vi "FRCts20_Backend_IssueTeamList.vi"(8 "error in (no error)":errorcluster) -> (0 "error out":errorcluster, 2 "IssueTeamList":T1)   [LabVIEW 2013, in "FRCts20_Backend_WebMethods.lvlib"]
doc: "The IssueTeamList function returns all teams with a currently open issue. It is sorted by open time longest to shortest. Caller is provided <b>Open time</b>, <b>Team Number</b>, <b>Loacation</b>, and <b>Description</b>."
uses:
  FRCts20_Backend_WebMethods.lvlib
  FRCts20_Backend_FGVOperation.ctl
  FRCts20_Backend_Engine.lvlib
  FRCts20_Backend_IssueTeamList.ctl
  FRCts20_Backend_Controls.lvlib
  FRCts20_Backend_request_info.ctl
  FRCts20_Backend_Note.ctl
  FRCts20_Backend_Note_list.ctl
  FRCts20_Backend_IssueDfn.ctl
panel:
  in  "IssueTeamList_Ref":T1
  # "The IssueTeamList function returns all teams with a\ncurrently open issue. It is sorted by open time longest \nto shortest. Caller is provided Open time, Team Number,\nLoacation, and Description."
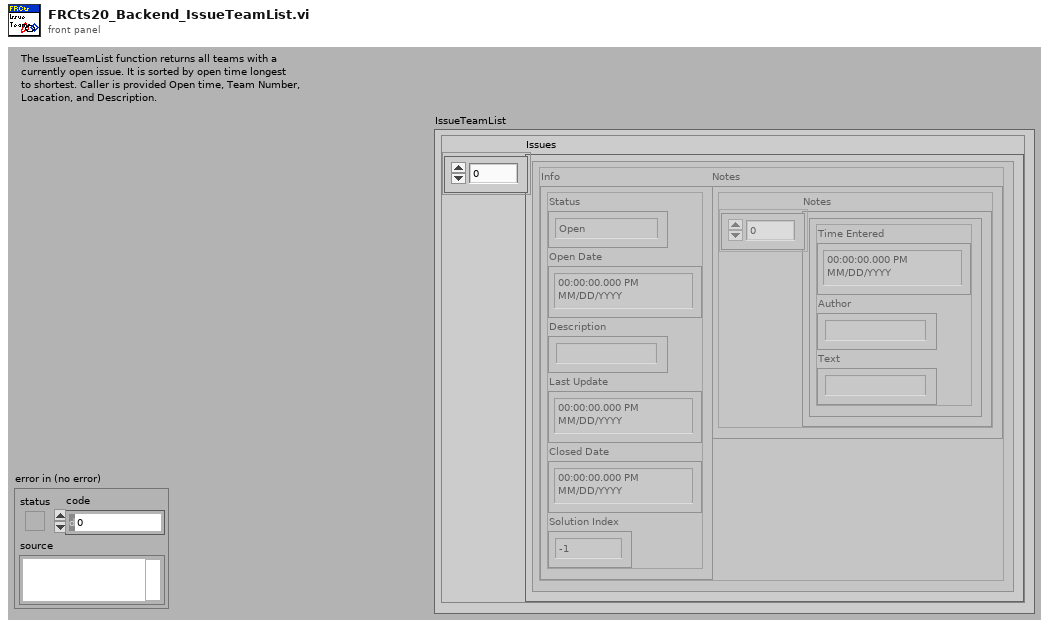
[diagram p1: front panel]
types:
  T1 = typedef "FRCts20_Backend_Controls.lvlib/FRCts20_Backend_IssueTeamList.ctl" = cluster{"Issues":T2[]}
  T2 = typedef "FRCts20_Backend_Controls.lvlib/FRCts20_Backend_IssueDfn.ctl" = cluster{"Notes":T3, "Info":T5}
  T3 = typedef "FRCts20_Backend_Controls.lvlib/FRCts20_Backend_Note_list.ctl" = cluster{"Notes":T4[]}
  T4 = typedef "FRCts20_Backend_Controls.lvlib/FRCts20_Backend_Note.ctl" = cluster{"Time Entered":timestamp, "Author":string, "Text":string}
  T5 = typedef "FRCts20_Backend_Controls.lvlib/FRCts20_Backend_request_info.ctl" = cluster{"Status":enum16{"Open", "In Work", "Closed"}, "Open Date":timestamp, "Description":string, "Last Update":timestamp, "Closed Date":timestamp, "Solution Index":i32}
  T6 = typedef "FRCts20_Backend_Engine.lvlib/FRCts20_Backend_FGVOperation.ctl" = enum16{"Initialize", "EnqueueMessage", "EnqueueDataReturn", "FlushMessage", "FlushDataReturn"}
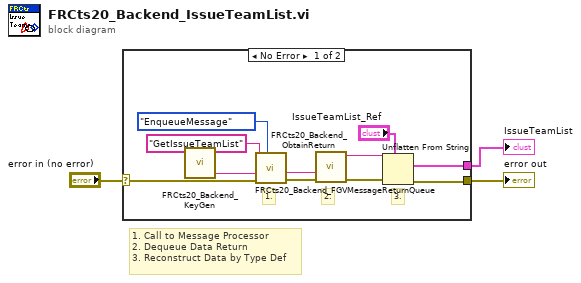
[diagram p0: block diagram]
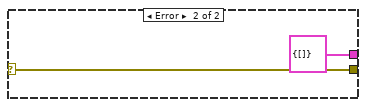
[diagram p2: hidden frame]
diagram:
  # "1. Call to Message Processor\n2. Dequeue Data Return\n3. Reconstruct Data by Type Def"
  n1 = case shown="No Error" "error in (no error)" {
    selector: "error in (no error)" -> [w14 w16]
    tunnel: [w8 w16] -> w2
    tunnel: [w6 T1 {"Issues"=[]} ("IssueTeamList_Ref")] -> w1
    frame No Error {
      # "3."
      # "2."
      # "1."
      n2 = call "FRCts20_Backend_KeyGen.vi"() -> ("Keygen"=w11:string)  [unwired: 27 in]
      n3 = call "FRCts20_Backend_FGVMessageReturnQueue.vi"("Operation"=FRCts20_Backend_FGVOperation."EnqueueMessage", "error in (no error)"=w14, "Key"=w11, "Message Name"="GetIssueTeamList") -> ("error out"=w10:errorcluster, "Key (Duplicate)"=w5:string)  [unwired: 4 in]
      n4 = call "FRCts20_Backend_ObtainReturn.vi"("error in (no error)"=w10, "Key"=w5) -> ("error out"=w9:errorcluster, "Message Value"=w4:string)  [unwired: 8 in]
      n5 = Unflatten From String(type="IssueTeamList_Ref", binary string=w4, error in (no error)=w9) -> (value=w6:T1, error out=w8:errorcluster)  [unwired: 2 in, 1 out]
    }
    frame Error {
    }
  }
  "error out" <- w2
  "IssueTeamList" <- w1
